vi "ShMemDescConstant.vi"() -> (0 "ShMemDesc 2":T1)   [LabVIEW 2009]
types:
  T1 = cluster{"NbrSamples":i32, "NbrRawSamples":i32, "NbrPeaks":i32, "NbrWaveforms":i32, "NbrSegments":i32, "NbrBlocks":i32, "NbrMemories":i32, "NbrBufs":i32, "NbrWrites":i32, "NbrRuns":i32, "iWaveform":i32, "iSegment":i32, "iBlock":i32, "iMemory":i32, "iBuf":i32, "iWrite":i32, "iRun":i32, "TotalBufsRecorded":i32, "TotalBufsProcessed":i32, "TotalBufsWritten":i32, "OverallBufsProcessed":i32, "TotalNbrMemories":i32, "TotalMemoriesProcessed":i32, "RawDataRecordedBuf1":u32, "RawDataRecordedBuf2":u32, "RawDataLastElementInBuffer1":u32, "RawDataLastElementInBuffer2":u32, "RawDataProcessedBuf1":u32, "RawDataProcessedBuf2":u32, "RawDataWrittenBuf1":u32, "RawDataWrittenBuf2":u32, "SampleInterval":sgl, "TofPeriod":i32, "dummy 3":i32, "BlockPeriod":i64, "BlockPulseDelay":i64, "BlockDelay":i64, "SingleIonSignal":sgl, "MassCalibMode":i32, "NbrMassCalibParams":i32, "dummy":i32, "p[16]":cluster{"[0]":dbl, "[1]":dbl, "[2]":dbl, "[3]":dbl, "[4]":dbl, "[5]":dbl, "[6]":dbl, "[7]":dbl, "[8]":dbl, "[9]":dbl, "[10]":dbl, "[11]":dbl, "[12]":dbl, "[13]":dbl, "[14]":dbl, "[15]":dbl}, "R0":sgl, "dm":sgl, "m0":sgl, "chIniFileName":cluster{"[0]":u8, "[1]":u8, "[2]":u8, "[3]":u8, "[4]":u8, "[5]":u8, "[6]":u8, "[7]":u8, "[8]":u8, "[9]":u8, "[10]":u8, "[11]":u8, "[12]":u8, "[13]":u8, "[14]":u8, "[15]":u8, "[16]":u8, "[17]":u8, "[18]":u8, "[19]":u8, "[20]":u8, "[21]":u8, "[22]":u8, "[23]":u8, "[24]":u8, "[25]":u8, "[26]":u8, "[27]":u8, "[28]":u8, "[29]":u8, "[30]":u8, "[31]":u8, "[32]":u8, "[33]":u8, "[34]":u8, "[35]":u8, "[36]":u8, "[37]":u8, "[38]":u8, "[39]":u8, "[40]":u8, "[41]":u8, "[42]":u8, "[43]":u8, "[44]":u8, "[45]":u8, "[46]":u8, "[47]":u8, "[48]":u8, "[49]":u8, "[50]":u8, "[51]":u8, "[52]":u8, "[53]":u8, "[54]":u8, "[55]":u8, "[56]":u8, "[57]":u8, "[58]":u8, "[59]":u8, "[60]":u8, "[61]":u8, "[62]":u8, "[63]":u8, "[64]":u8, "[65]":u8, "[66]":u8, "[67]":u8, "[68]":u8, "[69]":u8, "[70]":u8, "[71]":u8, "[72]":u8, "[73]":u8, "[74]":u8, "[75]":u8, "[76]":u8, "[77]":u8, "[78]":u8, "[79]":u8, "[80]":u8, "[81]":u8, "[82]":u8, "[83]":u8, "[84]":u8, "[85]":u8, "[86]":u8, "[87]":u8, "[88]":u8, "[89]":u8, "[90]":u8, "[91]":u8, "[92]":u8, "[93]":u8, "[94]":u8, "[95]":u8, "[96]":u8, "[97]":u8, "[98]":u8, "[99]":u8, "[100]":u8, "[101]":u8, "[102]":u8, "[103]":u8, "[104]":u8, "[105]":u8, "[106]":u8, "[107]":u8, "[108]":u8, "[109]":u8, "[110]":u8, "[111]":u8, "[112]":u8, "[113]":u8, "[114]":u8, "[115]":u8, "[116]":u8, "[117]":u8, "[118]":u8, "[119]":u8, "[120]":u8, "[121]":u8, "[122]":u8, "[123]":u8, "[124]":u8, "[125]":u8, "[126]":u8, "[127]":u8, "[128]":u8, "[129]":u8, "[130]":u8, "[131]":u8, "[132]":u8, "[133]":u8, "[134]":u8, "[135]":u8, "[136]":u8, "[137]":u8, "[138]":u8, "[139]":u8, "[140]":u8, "[141]":u8, "[142]":u8, "[143]":u8, "[144]":u8, "[145]":u8, "[146]":u8, "[147]":u8, "[148]":u8, "[149]":u8, "[150]":u8, "[151]":u8, "[152]":u8, "[153]":u8, "[154]":u8, "[155]":u8, "[156]":u8, "[157]":u8, "[158]":u8, "[159]":u8, "[160]":u8, "[161]":u8, "[162]":u8, "[163]":u8, "[164]":u8, "[165]":u8, "[166]":u8, "[167]":u8, "[168]":u8, "[169]":u8, "[170]":u8, "[171]":u8, "[172]":u8, "[173]":u8, "[174]":u8, "[175]":u8, "[176]":u8, "[177]":u8, "[178]":u8, "[179]":u8, "[180]":u8, "[181]":u8, "[182]":u8, "[183]":u8, "[184]":u8, "[185]":u8, "[186]":u8, "[187]":u8, "[188]":u8, "[189]":u8, "[190]":u8, "[191]":u8, "[192]":u8, "[193]":u8, "[194]":u8, "[195]":u8, "[196]":u8, "[197]":u8, "[198]":u8, "[199]":u8, "[200]":u8, "[201]":u8, "[202]":u8, "[203]":u8, "[204]":u8, "[205]":u8, "[206]":u8, "[207]":u8, "[208]":u8, "[209]":u8, "[210]":u8, "[211]":u8, "[212]":u8, "[213]":u8, "[214]":u8, "[215]":u8, "[216]":u8, "[217]":u8, "[218]":u8, "[219]":u8, "[220]":u8, "[221]":u8, "[222]":u8, "[223]":u8, "[224]":u8, "[225]":u8, "[226]":u8, "[227]":u8, "[228]":u8, "[229]":u8, "[230]":u8, "[231]":u8, "[232]":u8, "[233]":u8, "[234]":u8, "[235]":u8, "[236]":u8, "[237]":u8, "[238]":u8, "[239]":u8, "[240]":u8, "[241]":u8, "[242]":u8, "[243]":u8, "[244]":u8, "[245]":u8, "[246]":u8, "[247]":u8, "[248]":u8, "[249]":u8, "[250]":u8, "[251]":u8, "[252]":u8, "[253]":u8, "[254]":u8, "[255]":u8}, "CurrentDataFileName":cluster{"[0]":u8, "[1]":u8, "[2]":u8, "[3]":u8, "[4]":u8, "[5]":u8, "[6]":u8, "[7]":u8, "[8]":u8, "[9]":u8, "[10]":u8, "[11]":u8, "[12]":u8, "[13]":u8, "[14]":u8, "[15]":u8, "[16]":u8, "[17]":u8, "[18]":u8, "[19]":u8, "[20]":u8, "[21]":u8, "[22]":u8, "[23]":u8, "[24]":u8, "[25]":u8, "[26]":u8, "[27]":u8, "[28]":u8, "[29]":u8, "[30]":u8, "[31]":u8, "[32]":u8, "[33]":u8, "[34]":u8, "[35]":u8, "[36]":u8, "[37]":u8, "[38]":u8, "[39]":u8, "[40]":u8, "[41]":u8, "[42]":u8, "[43]":u8, "[44]":u8, "[45]":u8, "[46]":u8, "[47]":u8, "[48]":u8, "[49]":u8, "[50]":u8, "[51]":u8, "[52]":u8, "[53]":u8, "[54]":u8, "[55]":u8, "[56]":u8, "[57]":u8, "[58]":u8, "[59]":u8, "[60]":u8, "[61]":u8, "[62]":u8, "[63]":u8, "[64]":u8, "[65]":u8, "[66]":u8, "[67]":u8, "[68]":u8, "[69]":u8, "[70]":u8, "[71]":u8, "[72]":u8, "[73]":u8, "[74]":u8, "[75]":u8, "[76]":u8, "[77]":u8, "[78]":u8, "[79]":u8, "[80]":u8, "[81]":u8, "[82]":u8, "[83]":u8, "[84]":u8, "[85]":u8, "[86]":u8, "[87]":u8, "[88]":u8, "[89]":u8, "[90]":u8, "[91]":u8, "[92]":u8, "[93]":u8, "[94]":u8, "[95]":u8, "[96]":u8, "[97]":u8, "[98]":u8, "[99]":u8, "[100]":u8, "[101]":u8, "[102]":u8, "[103]":u8, "[104]":u8, "[105]":u8, "[106]":u8, "[107]":u8, "[108]":u8, "[109]":u8, "[110]":u8, "[111]":u8, "[112]":u8, "[113]":u8, "[114]":u8, "[115]":u8, "[116]":u8, "[117]":u8, "[118]":u8, "[119]":u8, "[120]":u8, "[121]":u8, "[122]":u8, "[123]":u8, "[124]":u8, "[125]":u8, "[126]":u8, "[127]":u8, "[128]":u8, "[129]":u8, "[130]":u8, "[131]":u8, "[132]":u8, "[133]":u8, "[134]":u8, "[135]":u8, "[136]":u8, "[137]":u8, "[138]":u8, "[139]":u8, "[140]":u8, "[141]":u8, "[142]":u8, "[143]":u8, "[144]":u8, "[145]":u8, "[146]":u8, "[147]":u8, "[148]":u8, "[149]":u8, "[150]":u8, "[151]":u8, "[152]":u8, "[153]":u8, "[154]":u8, "[155]":u8, "[156]":u8, "[157]":u8, "[158]":u8, "[159]":u8, "[160]":u8, "[161]":u8, "[162]":u8, "[163]":u8, "[164]":u8, "[165]":u8, "[166]":u8, "[167]":u8, "[168]":u8, "[169]":u8, "[170]":u8, "[171]":u8, "[172]":u8, "[173]":u8, "[174]":u8, "[175]":u8, "[176]":u8, "[177]":u8, "[178]":u8, "[179]":u8, "[180]":u8, "[181]":u8, "[182]":u8, "[183]":u8, "[184]":u8, "[185]":u8, "[186]":u8, "[187]":u8, "[188]":u8, "[189]":u8, "[190]":u8, "[191]":u8, "[192]":u8, "[193]":u8, "[194]":u8, "[195]":u8, "[196]":u8, "[197]":u8, "[198]":u8, "[199]":u8, "[200]":u8, "[201]":u8, "[202]":u8, "[203]":u8, "[204]":u8, "[205]":u8, "[206]":u8, "[207]":u8, "[208]":u8, "[209]":u8, "[210]":u8, "[211]":u8, "[212]":u8, "[213]":u8, "[214]":u8, "[215]":u8, "[216]":u8, "[217]":u8, "[218]":u8, "[219]":u8, "[220]":u8, "[221]":u8, "[222]":u8, "[223]":u8, "[224]":u8, "[225]":u8, "[226]":u8, "[227]":u8, "[228]":u8, "[229]":u8, "[230]":u8, "[231]":u8, "[232]":u8, "[233]":u8, "[234]":u8, "[235]":u8, "[236]":u8, "[237]":u8, "[238]":u8, "[239]":u8, "[240]":u8, "[241]":u8, "[242]":u8, "[243]":u8, "[244]":u8, "[245]":u8, "[246]":u8, "[247]":u8, "[248]":u8, "[249]":u8, "[250]":u8, "[251]":u8, "[252]":u8, "[253]":u8, "[254]":u8, "[255]":u8}, "DaqMode":i32, "AcquisitionMode":i32, "CombineMode":i32, "RecalibFreq":i32, "AcquisitionLogText":cluster{"[0]":u8, "[1]":u8, "[2]":u8, "[3]":u8, "[4]":u8, "[5]":u8, "[6]":u8, "[7]":u8, "[8]":u8, "[9]":u8, "[10]":u8, "[11]":u8, "[12]":u8, "[13]":u8, "[14]":u8, "[15]":u8, "[16]":u8, "[17]":u8, "[18]":u8, "[19]":u8, "[20]":u8, "[21]":u8, "[22]":u8, "[23]":u8, "[24]":u8, "[25]":u8, "[26]":u8, "[27]":u8, "[28]":u8, "[29]":u8, "[30]":u8, "[31]":u8, "[32]":u8, "[33]":u8, "[34]":u8, "[35]":u8, "[36]":u8, "[37]":u8, "[38]":u8, "[39]":u8, "[40]":u8, "[41]":u8, "[42]":u8, "[43]":u8, "[44]":u8, "[45]":u8, "[46]":u8, "[47]":u8, "[48]":u8, "[49]":u8, "[50]":u8, "[51]":u8, "[52]":u8, "[53]":u8, "[54]":u8, "[55]":u8, "[56]":u8, "[57]":u8, "[58]":u8, "[59]":u8, "[60]":u8, "[61]":u8, "[62]":u8, "[63]":u8, "[64]":u8, "[65]":u8, "[66]":u8, "[67]":u8, "[68]":u8, "[69]":u8, "[70]":u8, "[71]":u8, "[72]":u8, "[73]":u8, "[74]":u8, "[75]":u8, "[76]":u8, "[77]":u8, "[78]":u8, "[79]":u8, "[80]":u8, "[81]":u8, "[82]":u8, "[83]":u8, "[84]":u8, "[85]":u8, "[86]":u8, "[87]":u8, "[88]":u8, "[89]":u8, "[90]":u8, "[91]":u8, "[92]":u8, "[93]":u8, "[94]":u8, "[95]":u8, "[96]":u8, "[97]":u8, "[98]":u8, "[99]":u8, "[100]":u8, "[101]":u8, "[102]":u8, "[103]":u8, "[104]":u8, "[105]":u8, "[106]":u8, "[107]":u8, "[108]":u8, "[109]":u8, "[110]":u8, "[111]":u8, "[112]":u8, "[113]":u8, "[114]":u8, "[115]":u8, "[116]":u8, "[117]":u8, "[118]":u8, "[119]":u8, "[120]":u8, "[121]":u8, "[122]":u8, "[123]":u8, "[124]":u8, "[125]":u8, "[126]":u8, "[127]":u8, "[128]":u8, "[129]":u8, "[130]":u8, "[131]":u8, "[132]":u8, "[133]":u8, "[134]":u8, "[135]":u8, "[136]":u8, "[137]":u8, "[138]":u8, "[139]":u8, "[140]":u8, "[141]":u8, "[142]":u8, "[143]":u8, "[144]":u8, "[145]":u8, "[146]":u8, "[147]":u8, "[148]":u8, "[149]":u8, "[150]":u8, "[151]":u8, "[152]":u8, "[153]":u8, "[154]":u8, "[155]":u8, "[156]":u8, "[157]":u8, "[158]":u8, "[159]":u8, "[160]":u8, "[161]":u8, "[162]":u8, "[163]":u8, "[164]":u8, "[165]":u8, "[166]":u8, "[167]":u8, "[168]":u8, "[169]":u8, "[170]":u8, "[171]":u8, "[172]":u8, "[173]":u8, "[174]":u8, "[175]":u8, "[176]":u8, "[177]":u8, "[178]":u8, "[179]":u8, "[180]":u8, "[181]":u8, "[182]":u8, "[183]":u8, "[184]":u8, "[185]":u8, "[186]":u8, "[187]":u8, "[188]":u8, "[189]":u8, "[190]":u8, "[191]":u8, "[192]":u8, "[193]":u8, "[194]":u8, "[195]":u8, "[196]":u8, "[197]":u8, "[198]":u8, "[199]":u8, "[200]":u8, "[201]":u8, "[202]":u8, "[203]":u8, "[204]":u8, "[205]":u8, "[206]":u8, "[207]":u8, "[208]":u8, "[209]":u8, "[210]":u8, "[211]":u8, "[212]":u8, "[213]":u8, "[214]":u8, "[215]":u8, "[216]":u8, "[217]":u8, "[218]":u8, "[219]":u8, "[220]":u8, "[221]":u8, "[222]":u8, "[223]":u8, "[224]":u8, "[225]":u8, "[226]":u8, "[227]":u8, "[228]":u8, "[229]":u8, "[230]":u8, "[231]":u8, "[232]":u8, "[233]":u8, "[234]":u8, "[235]":u8, "[236]":u8, "[237]":u8, "[238]":u8, "[239]":u8, "[240]":u8, "[241]":u8, "[242]":u8, "[243]":u8, "[244]":u8, "[245]":u8, "[246]":u8, "[247]":u8, "[248]":u8, "[249]":u8, "[250]":u8, "[251]":u8, "[252]":u8, "[253]":u8, "[254]":u8, "[255]":u8}, "dummy 2":i32, "AcquisitionLogTime":u64, "TimeZero":u64, "ExternalLock":u32, "ProcessingLevel":u32, "AttributeType":i32, "AttributeObject":cluster{"[0]":u8, "[1]":u8, "[2]":u8, "[3]":u8, "[4]":u8, "[5]":u8, "[6]":u8, "[7]":u8, "[8]":u8, "[9]":u8, "[10]":u8, "[11]":u8, "[12]":u8, "[13]":u8, "[14]":u8, "[15]":u8, "[16]":u8, "[17]":u8, "[18]":u8, "[19]":u8, "[20]":u8, "[21]":u8, "[22]":u8, "[23]":u8, "[24]":u8, "[25]":u8, "[26]":u8, "[27]":u8, "[28]":u8, "[29]":u8, "[30]":u8, "[31]":u8, "[32]":u8, "[33]":u8, "[34]":u8, "[35]":u8, "[36]":u8, "[37]":u8, "[38]":u8, "[39]":u8, "[40]":u8, "[41]":u8, "[42]":u8, "[43]":u8, "[44]":u8, "[45]":u8, "[46]":u8, "[47]":u8, "[48]":u8, "[49]":u8, "[50]":u8, "[51]":u8, "[52]":u8, "[53]":u8, "[54]":u8, "[55]":u8, "[56]":u8, "[57]":u8, "[58]":u8, "[59]":u8, "[60]":u8, "[61]":u8, "[62]":u8, "[63]":u8, "[64]":u8, "[65]":u8, "[66]":u8, "[67]":u8, "[68]":u8, "[69]":u8, "[70]":u8, "[71]":u8, "[72]":u8, "[73]":u8, "[74]":u8, "[75]":u8, "[76]":u8, "[77]":u8, "[78]":u8, "[79]":u8, "[80]":u8, "[81]":u8, "[82]":u8, "[83]":u8, "[84]":u8, "[85]":u8, "[86]":u8, "[87]":u8, "[88]":u8, "[89]":u8, "[90]":u8, "[91]":u8, "[92]":u8, "[93]":u8, "[94]":u8, "[95]":u8, "[96]":u8, "[97]":u8, "[98]":u8, "[99]":u8, "[100]":u8, "[101]":u8, "[102]":u8, "[103]":u8, "[104]":u8, "[105]":u8, "[106]":u8, "[107]":u8, "[108]":u8, "[109]":u8, "[110]":u8, "[111]":u8, "[112]":u8, "[113]":u8, "[114]":u8, "[115]":u8, "[116]":u8, "[117]":u8, "[118]":u8, "[119]":u8, "[120]":u8, "[121]":u8, "[122]":u8, "[123]":u8, "[124]":u8, "[125]":u8, "[126]":u8, "[127]":u8, "[128]":u8, "[129]":u8, "[130]":u8, "[131]":u8, "[132]":u8, "[133]":u8, "[134]":u8, "[135]":u8, "[136]":u8, "[137]":u8, "[138]":u8, "[139]":u8, "[140]":u8, "[141]":u8, "[142]":u8, "[143]":u8, "[144]":u8, "[145]":u8, "[146]":u8, "[147]":u8, "[148]":u8, "[149]":u8, "[150]":u8, "[151]":u8, "[152]":u8, "[153]":u8, "[154]":u8, "[155]":u8, "[156]":u8, "[157]":u8, "[158]":u8, "[159]":u8, "[160]":u8, "[161]":u8, "[162]":u8, "[163]":u8, "[164]":u8, "[165]":u8, "[166]":u8, "[167]":u8, "[168]":u8, "[169]":u8, "[170]":u8, "[171]":u8, "[172]":u8, "[173]":u8, "[174]":u8, "[175]":u8, "[176]":u8, "[177]":u8, "[178]":u8, "[179]":u8, "[180]":u8, "[181]":u8, "[182]":u8, "[183]":u8, "[184]":u8, "[185]":u8, "[186]":u8, "[187]":u8, "[188]":u8, "[189]":u8, "[190]":u8, "[191]":u8, "[192]":u8, "[193]":u8, "[194]":u8, "[195]":u8, "[196]":u8, "[197]":u8, "[198]":u8, "[199]":u8, "[200]":u8, "[201]":u8, "[202]":u8, "[203]":u8, "[204]":u8, "[205]":u8, "[206]":u8, "[207]":u8, "[208]":u8, "[209]":u8, "[210]":u8, "[211]":u8, "[212]":u8, "[213]":u8, "[214]":u8, "[215]":u8, "[216]":u8, "[217]":u8, "[218]":u8, "[219]":u8, "[220]":u8, "[221]":u8, "[222]":u8, "[223]":u8, "[224]":u8, "[225]":u8, "[226]":u8, "[227]":u8, "[228]":u8, "[229]":u8, "[230]":u8, "[231]":u8, "[232]":u8, "[233]":u8, "[234]":u8, "[235]":u8, "[236]":u8, "[237]":u8, "[238]":u8, "[239]":u8, "[240]":u8, "[241]":u8, "[242]":u8, "[243]":u8, "[244]":u8, "[245]":u8, "[246]":u8, "[247]":u8, "[248]":u8, "[249]":u8, "[250]":u8, "[251]":u8, "[252]":u8, "[253]":u8, "[254]":u8, "[255]":u8}, "AttributeName":cluster{"[0]":u8, "[1]":u8, "[2]":u8, "[3]":u8, "[4]":u8, "[5]":u8, "[6]":u8, "[7]":u8, "[8]":u8, "[9]":u8, "[10]":u8, "[11]":u8, "[12]":u8, "[13]":u8, "[14]":u8, "[15]":u8, "[16]":u8, "[17]":u8, "[18]":u8, "[19]":u8, "[20]":u8, "[21]":u8, "[22]":u8, "[23]":u8, "[24]":u8, "[25]":u8, "[26]":u8, "[27]":u8, "[28]":u8, "[29]":u8, "[30]":u8, "[31]":u8, "[32]":u8, "[33]":u8, "[34]":u8, "[35]":u8, "[36]":u8, "[37]":u8, "[38]":u8, "[39]":u8, "[40]":u8, "[41]":u8, "[42]":u8, "[43]":u8, "[44]":u8, "[45]":u8, "[46]":u8, "[47]":u8, "[48]":u8, "[49]":u8, "[50]":u8, "[51]":u8, "[52]":u8, "[53]":u8, "[54]":u8, "[55]":u8, "[56]":u8, "[57]":u8, "[58]":u8, "[59]":u8, "[60]":u8, "[61]":u8, "[62]":u8, "[63]":u8, "[64]":u8, "[65]":u8, "[66]":u8, "[67]":u8, "[68]":u8, "[69]":u8, "[70]":u8, "[71]":u8, "[72]":u8, "[73]":u8, "[74]":u8, "[75]":u8, "[76]":u8, "[77]":u8, "[78]":u8, "[79]":u8, "[80]":u8, "[81]":u8, "[82]":u8, "[83]":u8, "[84]":u8, "[85]":u8, "[86]":u8, "[87]":u8, "[88]":u8, "[89]":u8, "[90]":u8, "[91]":u8, "[92]":u8, "[93]":u8, "[94]":u8, "[95]":u8, "[96]":u8, "[97]":u8, "[98]":u8, "[99]":u8, "[100]":u8, "[101]":u8, "[102]":u8, "[103]":u8, "[104]":u8, "[105]":u8, "[106]":u8, "[107]":u8, "[108]":u8, "[109]":u8, "[110]":u8, "[111]":u8, "[112]":u8, "[113]":u8, "[114]":u8, "[115]":u8, "[116]":u8, "[117]":u8, "[118]":u8, "[119]":u8, "[120]":u8, "[121]":u8, "[122]":u8, "[123]":u8, "[124]":u8, "[125]":u8, "[126]":u8, "[127]":u8}, "AttributeInt":i32, "AttributeDouble":dbl, "EnableVarNbrMemories":u32, "NbrSteps":i32, "CurrentStepAtBuf":i32, "NbrMemoriesForCurrentStep":i32}
diagram:
  "ShMemDesc 2" <- T1 {"NbrSamples"=0, "NbrRawSamples"=0, "NbrPeaks"=0, "NbrWaveforms"=0, "NbrSegments"=0, "NbrBlocks"=0, "NbrMemories"=0, "NbrBufs"=0, "NbrWrites"=0, "NbrRuns"=0, "iWaveform"=0, "iSegment"=0, "iBlock"=0, "iMemory"=0, "iBuf"=0, "iWrite"=0, "iRun"=0, "TotalBufsRecorded"=0, "TotalBufsProcessed"=0, "TotalBufsWritten"=0, "OverallBufsProcessed"=0, "TotalNbrMemories"=0, "TotalMemoriesProcessed"=0, "RawDataRecordedBuf1"=0, "RawDataRecordedBuf2"=0, "RawDataLastElementInBuffer1"=0, "RawDataLastElementInBuffer2"=0, "RawDataProcessedBuf1"=0, "RawDataProcessedBuf2"=0, "RawDataWrittenBuf1"=0, "RawDataWrittenBuf2"=0, "SampleInterval"=0.0, "TofPeriod"=0, "dummy 3"=0, "BlockPeriod"=0, "BlockPulseDelay"=0, "BlockDelay"=0, "SingleIonSignal"=0.0, "MassCalibMode"=0, "NbrMassCalibParams"=0, "dummy"=0, "p[16]"={"[0]"=0.0, "[1]"=0.0, "[2]"=0.0, "[3]"=0.0, "[4]"=0.0, "[5]"=0.0, "[6]"=0.0, "[7]"=0.0, "[8]"=0.0, "[9]"=0.0, "[10]"=0.0, "[11]"=0.0, "[12]"=0.0, "[13]"=0.0, "[14]"=0.0, "[15]"=0.0}, "R0"=0.0, "dm"=0.0, "m0"=0.0, "chIniFileName"={"[0]"=0, "[1]"=0, "[2]"=0, "[3]"=0, "[4]"=0, "[5]"=0, "[6]"=0, "[7]"=0, "[8]"=0, "[9]"=0, "[10]"=0, "[11]"=0, "[12]"=0, "[13]"=0, "[14]"=0, "[15]"=0, "[16]"=0, "[17]"=0, "[18]"=0, "[19]"=0, "[20]"=0, "[21]"=0, "[22]"=0, "[23]"=0, "[24]"=0, "[25]"=0, "[26]"=0, "[27]"=0, "[28]"=0, "[29]"=0, "[30]"=0, "[31]"=0, "[32]"=0, "[33]"=0, "[34]"=0, "[35]"=0, "[36]"=0, "[37]"=0, "[38]"=0, "[39]"=0, "[40]"=0, "[41]"=0, "[42]"=0, "[43]"=0, "[44]"=0, "[45]"=0, "[46]"=0, "[47]"=0, "[48]"=0, "[49]"=0, "[50]"=0, "[51]"=0, "[52]"=0, "[53]"=0, "[54]"=0, "[55]"=0, "[56]"=0, "[57]"=0, "[58]"=0, "[59]"=0, "[60]"=0, "[61]"=0, "[62]"=0, "[63]"=0, "[64]"=0, "[65]"=0, "[66]"=0, "[67]"=0, "[68]"=0, "[69]"=0, "[70]"=0, "[71]"=0, "[72]"=0, "[73]"=0, "[74]"=0, "[75]"=0, "[76]"=0, "[77]"=0, "[78]"=0, "[79]"=0, "[80]"=0, "[81]"=0, "[82]"=0, "[83]"=0, "[84]"=0, "[85]"=0, "[86]"=0, "[87]"=0, "[88]"=0, "[89]"=0, "[90]"=0, "[91]"=0, "[92]"=0, "[93]"=0, "[94]"=0, "[95]"=0, "[96]"=0, "[97]"=0, "[98]"=0, "[99]"=0, "[100]"=0, "[101]"=0, "[102]"=0, "[103]"=0, "[104]"=0, "[105]"=0, "[106]"=0, "[107]"=0, "[108]"=0, "[109]"=0, "[110]"=0, "[111]"=0, "[112]"=0, "[113]"=0, "[114]"=0, "[115]"=0, "[116]"=0, "[117]"=0, "[118]"=0, "[119]"=0, "[120]"=0, "[121]"=0, "[122]"=0, "[123]"=0, "[124]"=0, "[125]"=0, "[126]"=0, "[127]"=0, "[128]"=0, "[129]"=0, "[130]"=0, "[131]"=0, "[132]"=0, "[133]"=0, "[134]"=0, "[135]"=0, "[136]"=0, "[137]"=0, "[138]"=0, "[139]"=0, "[140]"=0, "[141]"=0, "[142]"=0, "[143]"=0, "[144]"=0, "[145]"=0, "[146]"=0, "[147]"=0, "[148]"=0, "[149]"=0, "[150]"=0, "[151]"=0, "[152]"=0, "[153]"=0, "[154]"=0, "[155]"=0, "[156]"=0, "[157]"=0, "[158]"=0, "[159]"=0, "[160]"=0, "[161]"=0, "[162]"=0, "[163]"=0, "[164]"=0, "[165]"=0, "[166]"=0, "[167]"=0, "[168]"=0, "[169]"=0, "[170]"=0, "[171]"=0, "[172]"=0, "[173]"=0, "[174]"=0, "[175]"=0, "[176]"=0, "[177]"=0, "[178]"=0, "[179]"=0, "[180]"=0, "[181]"=0, "[182]"=0, "[183]"=0, "[184]"=0, "[185]"=0, "[186]"=0, "[187]"=0, "[188]"=0, "[189]"=0, "[190]"=0, "[191]"=0, "[192]"=0, "[193]"=0, "[194]"=0, "[195]"=0, "[196]"=0, "[197]"=0, "[198]"=0, "[199]"=0, "[200]"=0, "[201]"=0, "[202]"=0, "[203]"=0, "[204]"=0, "[205]"=0, "[206]"=0, "[207]"=0, "[208]"=0, "[209]"=0, "[210]"=0, "[211]"=0, "[212]"=0, "[213]"=0, "[214]"=0, "[215]"=0, "[216]"=0, "[217]"=0, "[218]"=0, "[219]"=0, "[220]"=0, "[221]"=0, "[222]"=0, "[223]"=0, "[224]"=0, "[225]"=0, "[226]"=0, "[227]"=0, "[228]"=0, "[229]"=0, "[230]"=0, "[231]"=0, "[232]"=0, "[233]"=0, "[234]"=0, "[235]"=0, "[236]"=0, "[237]"=0, "[238]"=0, "[239]"=0, "[240]"=0, "[241]"=0, "[242]"=0, "[243]"=0, "[244]"=0, "[245]"=0, "[246]"=0, "[247]"=0, "[248]"=0, "[249]"=0, "[250]"=0, "[251]"=0, "[252]"=0, "[253]"=0, "[254]"=0, "[255]"=0}, "CurrentDataFileName"={"[0]"=0, "[1]"=0, "[2]"=0, "[3]"=0, "[4]"=0, "[5]"=0, "[6]"=0, "[7]"=0, "[8]"=0, "[9]"=0, "[10]"=0, "[11]"=0, "[12]"=0, "[13]"=0, "[14]"=0, "[15]"=0, "[16]"=0, "[17]"=0, "[18]"=0, "[19]"=0, "[20]"=0, "[21]"=0, "[22]"=0, "[23]"=0, "[24]"=0, "[25]"=0, "[26]"=0, "[27]"=0, "[28]"=0, "[29]"=0, "[30]"=0, "[31]"=0, "[32]"=0, "[33]"=0, "[34]"=0, "[35]"=0, "[36]"=0, "[37]"=0, "[38]"=0, "[39]"=0, "[40]"=0, "[41]"=0, "[42]"=0, "[43]"=0, "[44]"=0, "[45]"=0, "[46]"=0, "[47]"=0, "[48]"=0, "[49]"=0, "[50]"=0, "[51]"=0, "[52]"=0, "[53]"=0, "[54]"=0, "[55]"=0, "[56]"=0, "[57]"=0, "[58]"=0, "[59]"=0, "[60]"=0, "[61]"=0, "[62]"=0, "[63]"=0, "[64]"=0, "[65]"=0, "[66]"=0, "[67]"=0, "[68]"=0, "[69]"=0, "[70]"=0, "[71]"=0, "[72]"=0, "[73]"=0, "[74]"=0, "[75]"=0, "[76]"=0, "[77]"=0, "[78]"=0, "[79]"=0, "[80]"=0, "[81]"=0, "[82]"=0, "[83]"=0, "[84]"=0, "[85]"=0, "[86]"=0, "[87]"=0, "[88]"=0, "[89]"=0, "[90]"=0, "[91]"=0, "[92]"=0, "[93]"=0, "[94]"=0, "[95]"=0, "[96]"=0, "[97]"=0, "[98]"=0, "[99]"=0, "[100]"=0, "[101]"=0, "[102]"=0, "[103]"=0, "[104]"=0, "[105]"=0, "[106]"=0, "[107]"=0, "[108]"=0, "[109]"=0, "[110]"=0, "[111]"=0, "[112]"=0, "[113]"=0, "[114]"=0, "[115]"=0, "[116]"=0, "[117]"=0, "[118]"=0, "[119]"=0, "[120]"=0, "[121]"=0, "[122]"=0, "[123]"=0, "[124]"=0, "[125]"=0, "[126]"=0, "[127]"=0, "[128]"=0, "[129]"=0, "[130]"=0, "[131]"=0, "[132]"=0, "[133]"=0, "[134]"=0, "[135]"=0, "[136]"=0, "[137]"=0, "[138]"=0, "[139]"=0, "[140]"=0, "[141]"=0, "[142]"=0, "[143]"=0, "[144]"=0, "[145]"=0, "[146]"=0, "[147]"=0, "[148]"=0, "[149]"=0, "[150]"=0, "[151]"=0, "[152]"=0, "[153]"=0, "[154]"=0, "[155]"=0, "[156]"=0, "[157]"=0, "[158]"=0, "[159]"=0, "[160]"=0, "[161]"=0, "[162]"=0, "[163]"=0, "[164]"=0, "[165]"=0, "[166]"=0, "[167]"=0, "[168]"=0, "[169]"=0, "[170]"=0, "[171]"=0, "[172]"=0, "[173]"=0, "[174]"=0, "[175]"=0, "[176]"=0, "[177]"=0, "[178]"=0, "[179]"=0, "[180]"=0, "[181]"=0, "[182]"=0, "[183]"=0, "[184]"=0, "[185]"=0, "[186]"=0, "[187]"=0, "[188]"=0, "[189]"=0, "[190]"=0, "[191]"=0, "[192]"=0, "[193]"=0, "[194]"=0, "[195]"=0, "[196]"=0, "[197]"=0, "[198]"=0, "[199]"=0, "[200]"=0, "[201]"=0, "[202]"=0, "[203]"=0, "[204]"=0, "[205]"=0, "[206]"=0, "[207]"=0, "[208]"=0, "[209]"=0, "[210]"=0, "[211]"=0, "[212]"=0, "[213]"=0, "[214]"=0, "[215]"=0, "[216]"=0, "[217]"=0, "[218]"=0, "[219]"=0, "[220]"=0, "[221]"=0, "[222]"=0, "[223]"=0, "[224]"=0, "[225]"=0, "[226]"=0, "[227]"=0, "[228]"=0, "[229]"=0, "[230]"=0, "[231]"=0, "[232]"=0, "[233]"=0, "[234]"=0, "[235]"=0, "[236]"=0, "[237]"=0, "[238]"=0, "[239]"=0, "[240]"=0, "[241]"=0, "[242]"=0, "[243]"=0, "[244]"=0, "[245]"=0, "[246]"=0, "[247]"=0, "[248]"=0, "[249]"=0, "[250]"=0, "[251]"=0, "[252]"=0, "[253]"=0, "[254]"=0, "[255]"=0}, "DaqMode"=0, "AcquisitionMode"=0, "CombineMode"=0, "RecalibFreq"=0, "AcquisitionLogText"={"[0]"=0, "[1]"=0, "[2]"=0, "[3]"=0, "[4]"=0, "[5]"=0, "[6]"=0, "[7]"=0, "[8]"=0, "[9]"=0, "[10]"=0, "[11]"=0, "[12]"=0, "[13]"=0, "[14]"=0, "[15]"=0, "[16]"=0, "[17]"=0, "[18]"=0, "[19]"=0, "[20]"=0, "[21]"=0, "[22]"=0, "[23]"=0, "[24]"=0, "[25]"=0, "[26]"=0, "[27]"=0, "[28]"=0, "[29]"=0, "[30]"=0, "[31]"=0, "[32]"=0, "[33]"=0, "[34]"=0, "[35]"=0, "[36]"=0, "[37]"=0, "[38]"=0, "[39]"=0, "[40]"=0, "[41]"=0, "[42]"=0, "[43]"=0, "[44]"=0, "[45]"=0, "[46]"=0, "[47]"=0, "[48]"=0, "[49]"=0, "[50]"=0, "[51]"=0, "[52]"=0, "[53]"=0, "[54]"=0, "[55]"=0, "[56]"=0, "[57]"=0, "[58]"=0, "[59]"=0, "[60]"=0, "[61]"=0, "[62]"=0, "[63]"=0, "[64]"=0, "[65]"=0, "[66]"=0, "[67]"=0, "[68]"=0, "[69]"=0, "[70]"=0, "[71]"=0, "[72]"=0, "[73]"=0, "[74]"=0, "[75]"=0, "[76]"=0, "[77]"=0, "[78]"=0, "[79]"=0, "[80]"=0, "[81]"=0, "[82]"=0, "[83]"=0, "[84]"=0, "[85]"=0, "[86]"=0, "[87]"=0, "[88]"=0, "[89]"=0, "[90]"=0, "[91]"=0, "[92]"=0, "[93]"=0, "[94]"=0, "[95]"=0, "[96]"=0, "[97]"=0, "[98]"=0, "[99]"=0, "[100]"=0, "[101]"=0, "[102]"=0, "[103]"=0, "[104]"=0, "[105]"=0, "[106]"=0, "[107]"=0, "[108]"=0, "[109]"=0, "[110]"=0, "[111]"=0, "[112]"=0, "[113]"=0, "[114]"=0, "[115]"=0, "[116]"=0, "[117]"=0, "[118]"=0, "[119]"=0, "[120]"=0, "[121]"=0, "[122]"=0, "[123]"=0, "[124]"=0, "[125]"=0, "[126]"=0, "[127]"=0, "[128]"=0, "[129]"=0, "[130]"=0, "[131]"=0, "[132]"=0, "[133]"=0, "[134]"=0, "[135]"=0, "[136]"=0, "[137]"=0, "[138]"=0, "[139]"=0, "[140]"=0, "[141]"=0, "[142]"=0, "[143]"=0, "[144]"=0, "[145]"=0, "[146]"=0, "[147]"=0, "[148]"=0, "[149]"=0, "[150]"=0, "[151]"=0, "[152]"=0, "[153]"=0, "[154]"=0, "[155]"=0, "[156]"=0, "[157]"=0, "[158]"=0, "[159]"=0, "[160]"=0, "[161]"=0, "[162]"=0, "[163]"=0, "[164]"=0, "[165]"=0, "[166]"=0, "[167]"=0, "[168]"=0, "[169]"=0, "[170]"=0, "[171]"=0, "[172]"=0, "[173]"=0, "[174]"=0, "[175]"=0, "[176]"=0, "[177]"=0, "[178]"=0, "[179]"=0, "[180]"=0, "[181]"=0, "[182]"=0, "[183]"=0, "[184]"=0, "[185]"=0, "[186]"=0, "[187]"=0, "[188]"=0, "[189]"=0, "[190]"=0, "[191]"=0, "[192]"=0, "[193]"=0, "[194]"=0, "[195]"=0, "[196]"=0, "[197]"=0, "[198]"=0, "[199]"=0, "[200]"=0, "[201]"=0, "[202]"=0, "[203]"=0, "[204]"=0, "[205]"=0, "[206]"=0, "[207]"=0, "[208]"=0, "[209]"=0, "[210]"=0, "[211]"=0, "[212]"=0, "[213]"=0, "[214]"=0, "[215]"=0, "[216]"=0, "[217]"=0, "[218]"=0, "[219]"=0, "[220]"=0, "[221]"=0, "[222]"=0, "[223]"=0, "[224]"=0, "[225]"=0, "[226]"=0, "[227]"=0, "[228]"=0, "[229]"=0, "[230]"=0, "[231]"=0, "[232]"=0, "[233]"=0, "[234]"=0, "[235]"=0, "[236]"=0, "[237]"=0, "[238]"=0, "[239]"=0, "[240]"=0, "[241]"=0, "[242]"=0, "[243]"=0, "[244]"=0, "[245]"=0, "[246]"=0, "[247]"=0, "[248]"=0, "[249]"=0, "[250]"=0, "[251]"=0, "[252]"=0, "[253]"=0, "[254]"=0, "[255]"=0}, "dummy 2"=0, "AcquisitionLogTime"=0, "TimeZero"=0, "ExternalLock"=0, "ProcessingLevel"=0, "AttributeType"=0, "AttributeObject"={"[0]"=0, "[1]"=0, "[2]"=0, "[3]"=0, "[4]"=0, "[5]"=0, "[6]"=0, "[7]"=0, "[8]"=0, "[9]"=0, "[10]"=0, "[11]"=0, "[12]"=0, "[13]"=0, "[14]"=0, "[15]"=0, "[16]"=0, "[17]"=0, "[18]"=0, "[19]"=0, "[20]"=0, "[21]"=0, "[22]"=0, "[23]"=0, "[24]"=0, "[25]"=0, "[26]"=0, "[27]"=0, "[28]"=0, "[29]"=0, "[30]"=0, "[31]"=0, "[32]"=0, "[33]"=0, "[34]"=0, "[35]"=0, "[36]"=0, "[37]"=0, "[38]"=0, "[39]"=0, "[40]"=0, "[41]"=0, "[42]"=0, "[43]"=0, "[44]"=0, "[45]"=0, "[46]"=0, "[47]"=0, "[48]"=0, "[49]"=0, "[50]"=0, "[51]"=0, "[52]"=0, "[53]"=0, "[54]"=0, "[55]"=0, "[56]"=0, "[57]"=0, "[58]"=0, "[59]"=0, "[60]"=0, "[61]"=0, "[62]"=0, "[63]"=0, "[64]"=0, "[65]"=0, "[66]"=0, "[67]"=0, "[68]"=0, "[69]"=0, "[70]"=0, "[71]"=0, "[72]"=0, "[73]"=0, "[74]"=0, "[75]"=0, "[76]"=0, "[77]"=0, "[78]"=0, "[79]"=0, "[80]"=0, "[81]"=0, "[82]"=0, "[83]"=0, "[84]"=0, "[85]"=0, "[86]"=0, "[87]"=0, "[88]"=0, "[89]"=0, "[90]"=0, "[91]"=0, "[92]"=0, "[93]"=0, "[94]"=0, "[95]"=0, "[96]"=0, "[97]"=0, "[98]"=0, "[99]"=0, "[100]"=0, "[101]"=0, "[102]"=0, "[103]"=0, "[104]"=0, "[105]"=0, "[106]"=0, "[107]"=0, "[108]"=0, "[109]"=0, "[110]"=0, "[111]"=0, "[112]"=0, "[113]"=0, "[114]"=0, "[115]"=0, "[116]"=0, "[117]"=0, "[118]"=0, "[119]"=0, "[120]"=0, "[121]"=0, "[122]"=0, "[123]"=0, "[124]"=0, "[125]"=0, "[126]"=0, "[127]"=0, "[128]"=0, "[129]"=0, "[130]"=0, "[131]"=0, "[132]"=0, "[133]"=0, "[134]"=0, "[135]"=0, "[136]"=0, "[137]"=0, "[138]"=0, "[139]"=0, "[140]"=0, "[141]"=0, "[142]"=0, "[143]"=0, "[144]"=0, "[145]"=0, "[146]"=0, "[147]"=0, "[148]"=0, "[149]"=0, "[150]"=0, "[151]"=0, "[152]"=0, "[153]"=0, "[154]"=0, "[155]"=0, "[156]"=0, "[157]"=0, "[158]"=0, "[159]"=0, "[160]"=0, "[161]"=0, "[162]"=0, "[163]"=0, "[164]"=0, "[165]"=0, "[166]"=0, "[167]"=0, "[168]"=0, "[169]"=0, "[170]"=0, "[171]"=0, "[172]"=0, "[173]"=0, "[174]"=0, "[175]"=0, "[176]"=0, "[177]"=0, "[178]"=0, "[179]"=0, "[180]"=0, "[181]"=0, "[182]"=0, "[183]"=0, "[184]"=0, "[185]"=0, "[186]"=0, "[187]"=0, "[188]"=0, "[189]"=0, "[190]"=0, "[191]"=0, "[192]"=0, "[193]"=0, "[194]"=0, "[195]"=0, "[196]"=0, "[197]"=0, "[198]"=0, "[199]"=0, "[200]"=0, "[201]"=0, "[202]"=0, "[203]"=0, "[204]"=0, "[205]"=0, "[206]"=0, "[207]"=0, "[208]"=0, "[209]"=0, "[210]"=0, "[211]"=0, "[212]"=0, "[213]"=0, "[214]"=0, "[215]"=0, "[216]"=0, "[217]"=0, "[218]"=0, "[219]"=0, "[220]"=0, "[221]"=0, "[222]"=0, "[223]"=0, "[224]"=0, "[225]"=0, "[226]"=0, "[227]"=0, "[228]"=0, "[229]"=0, "[230]"=0, "[231]"=0, "[232]"=0, "[233]"=0, "[234]"=0, "[235]"=0, "[236]"=0, "[237]"=0, "[238]"=0, "[239]"=0, "[240]"=0, "[241]"=0, "[242]"=0, "[243]"=0, "[244]"=0, "[245]"=0, "[246]"=0, "[247]"=0, "[248]"=0, "[249]"=0, "[250]"=0, "[251]"=0, "[252]"=0, "[253]"=0, "[254]"=0, "[255]"=0}, "AttributeName"={"[0]"=0, "[1]"=0, "[2]"=0, "[3]"=0, "[4]"=0, "[5]"=0, "[6]"=0, "[7]"=0, "[8]"=0, "[9]"=0, "[10]"=0, "[11]"=0, "[12]"=0, "[13]"=0, "[14]"=0, "[15]"=0, "[16]"=0, "[17]"=0, "[18]"=0, "[19]"=0, "[20]"=0, "[21]"=0, "[22]"=0, "[23]"=0, "[24]"=0, "[25]"=0, "[26]"=0, "[27]"=0, "[28]"=0, "[29]"=0, "[30]"=0, "[31]"=0, "[32]"=0, "[33]"=0, "[34]"=0, "[35]"=0, "[36]"=0, "[37]"=0, "[38]"=0, "[39]"=0, "[40]"=0, "[41]"=0, "[42]"=0, "[43]"=0, "[44]"=0, "[45]"=0, "[46]"=0, "[47]"=0, "[48]"=0, "[49]"=0, "[50]"=0, "[51]"=0, "[52]"=0, "[53]"=0, "[54]"=0, "[55]"=0, "[56]"=0, "[57]"=0, "[58]"=0, "[59]"=0, "[60]"=0, "[61]"=0, "[62]"=0, "[63]"=0, "[64]"=0, "[65]"=0, "[66]"=0, "[67]"=0, "[68]"=0, "[69]"=0, "[70]"=0, "[71]"=0, "[72]"=0, "[73]"=0, "[74]"=0, "[75]"=0, "[76]"=0, "[77]"=0, "[78]"=0, "[79]"=0, "[80]"=0, "[81]"=0, "[82]"=0, "[83]"=0, "[84]"=0, "[85]"=0, "[86]"=0, "[87]"=0, "[88]"=0, "[89]"=0, "[90]"=0, "[91]"=0, "[92]"=0, "[93]"=0, "[94]"=0, "[95]"=0, "[96]"=0, "[97]"=0, "[98]"=0, "[99]"=0, "[100]"=0, "[101]"=0, "[102]"=0, "[103]"=0, "[104]"=0, "[105]"=0, "[106]"=0, "[107]"=0, "[108]"=0, "[109]"=0, "[110]"=0, "[111]"=0, "[112]"=0, "[113]"=0, "[114]"=0, "[115]"=0, "[116]"=0, "[117]"=0, "[118]"=0, "[119]"=0, "[120]"=0, "[121]"=0, "[122]"=0, "[123]"=0, "[124]"=0, "[125]"=0, "[126]"=0, "[127]"=0}, "AttributeInt"=0, "AttributeDouble"=0.0, "EnableVarNbrMemories"=0, "NbrSteps"=0, "CurrentStepAtBuf"=0, "NbrMemoriesForCurrentStep"=0} ("ShMemDesc 2")
